vi "Generate DAQ Waveform.vi"(4 "Debug Message FIFO":refnum<k33>, 7 "DAQ Config Data":T1, 8 "error in (no error)":errorcluster, 9 "Channel Data":dbl[](array[numeric]), 10 "Phase Array In":dbl[](array[numeric])) -> (0 "error out":errorcluster, 3 "Waveform Array":waveform(dbl)[](array[waveform]), 5 "Phase Array Out out":dbl[](array[numeric]))   [LabVIEW 2023, in "Waveform Analog Output Engine.lvlib"]
doc: "Create an array of waveforms based on the channel settings from the VeriStand engine"
uses:
  Waveform Analog Output Engine.lvlib
  DAQ Config Data.ctl
  <vilib>/measure/NI_MABase.lvlib
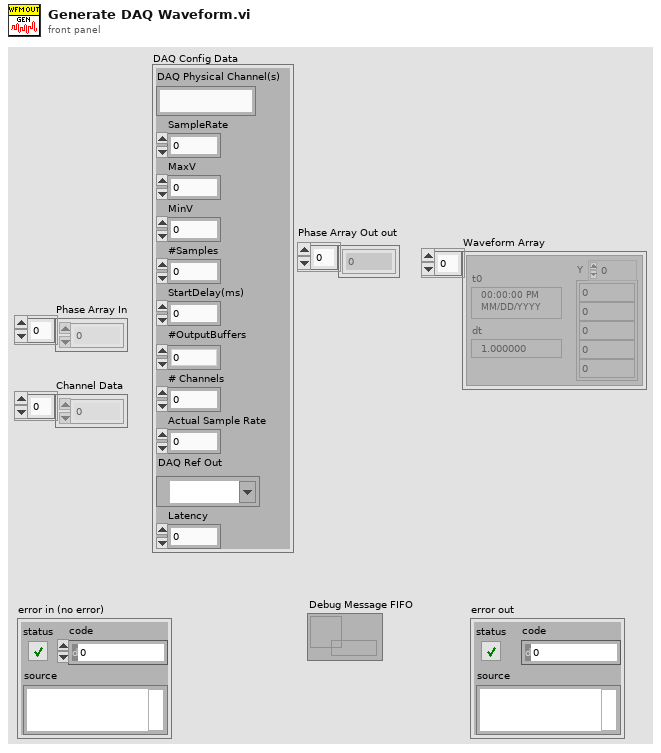
[diagram p1: front panel]
types:
  T1 = typedef "Waveform Analog Output Engine.lvlib/DAQ Config Data.ctl" = cluster{"DAQ Physical Channel(s)":string, "SampleRate":dbl, "MaxV":dbl, "MinV":dbl, "#Samples":dbl, "StartDelay(ms)":dbl, "#OutputBuffers":dbl, "# Channels":i32, "Actual Sample Rate":dbl, "DAQ Ref Out":refnum<k21>, "Latency":dbl}
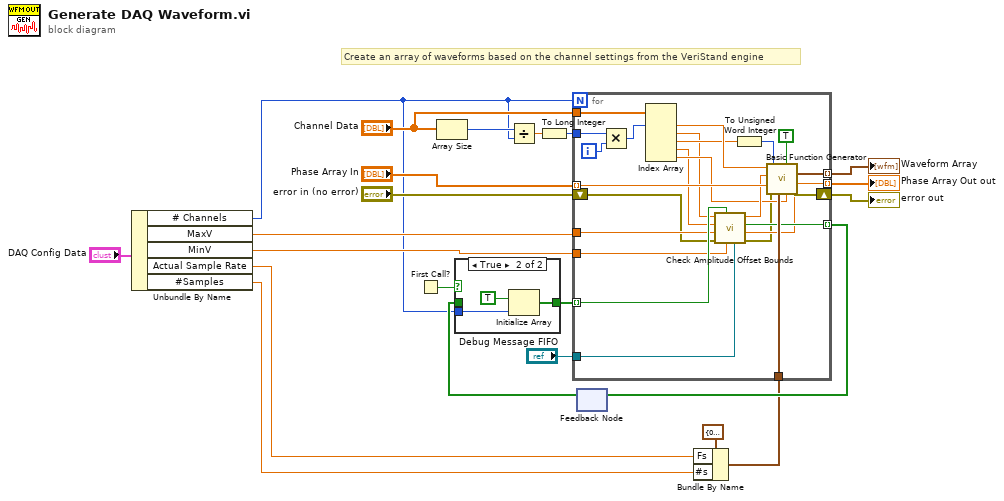
[diagram p0: block diagram]
diagram:
  # "Create an array of waveforms based on the channel settings from the VeriStand engine"
  n1 = Unbundle By Name("DAQ Config Data") -> ("# Channels"=w1:i32, "MaxV"=w10:dbl, "MinV"=w9:dbl, "Actual Sample Rate"=w4:dbl, "#Samples"=w3:dbl)
  n2 = First Call?() -> (First Call?: T/F=w13:bool)
  n3 = Array Size(array="Channel Data") -> (size(s)=w20:i32)
  n4 = Divide(x=w20, y=w1) -> (x/y=w21:dbl)
  n5 = To Long Integer(number=w21) -> (32bit integer=w22:i32)
  n6 = feedback #1() -> (w7:bool[])  [unwired: 1 in]
  n7 = case shown="True" w13 {
    tunnel: w1 -> [_ w26]
    tunnel: [w23 w24] -> w12
    tunnel: w7 -> [w23 _]
    frame False {
    }
    frame True {
      n8 = Initialize Array(TRUE, w26) -> (w24:bool[])
    }
  }
  n9 = Bundle By Name(cluster=cluster{"Fs":dbl, "#s":dbl} {"Fs"=0.0, "#s"=0.0} ("sampling info"), "Fs"=w4, "#s"=w3) -> (w2:cluster{"Fs":dbl, "#s":dbl})
  n10 = for {
    N: w1 -> [_]
    tunnel: w2 -> [w51]
    tunnel: [w50] -> w14 mode=indexing
    tunnel: [w49] -> w16 mode=indexing
    tunnel: "Phase Array In" -> [w48] mode=indexing
    shift-right: [w47] -> w18
    shift-left: "error in (no error)" -> [w30]
    tunnel: "Channel Data" -> [w46]
    tunnel: w22 -> [w40]
    tunnel: w12 -> [w38] mode=indexing
    tunnel: w10 -> [w34]
    tunnel: w9 -> [w35]
    tunnel: [w37] -> w8 mode=indexing
    tunnel: "Debug Message FIFO" -> [w28]
    i -> [w45]
    n11 = Multiply(x=w40, y=w45) -> (x*y=w44:i32)
    n12 = Index Array(array=w46, index #1=w44) -> (element #1=w43:dbl, element #2=w27:dbl, element #3=w42:dbl, element #4=w32:dbl, element #5=w33:dbl)  [unwired: 4 in]
    n13 = call "Check Amplitude Offset Bounds.vi"("Debug Message FIFO"=w28, "MinV"=w35, "Last Iter In Bounds?"=w38, "error in (no error)"=w30, "MaxV"=w34, "Offset"=w32, "Amplitude"=w27) -> ("error out"=w29:errorcluster, "Coerced Offset"=w31:dbl, "Values In Bounds?"=w37:bool, "Coerced Amplitude"=w36:dbl)  [unwired: 1 in]
    n14 = To Unsigned Word Integer(number=w42) -> (unsigned 16bit integer=w41:u16)
    n15 = call <vilib>:"Basic Function Generator.vi"("offset"=w31, "square wave duty cycle (%)"=w33, "reset signal"=TRUE, "sampling info"=w51, "signal type"=w41, "error in (no error)"=w29, "phase"=w48, "amplitude"=w36, "frequency"=w43) -> ("error out"=w47:errorcluster, "phase out"=w49:dbl, "signal out"=w50:waveform(dbl))
  }
  "error out" <- w18
  "Phase Array Out out" <- w16
  "Waveform Array" <- w14
  n16 = feedback-in #1(w8) -> ()
